vi "运维调试_采配水_古田户外.vi"() -> ()   [LabVIEW 2016, in "PLC.lvlib"]
uses:
  PLC.lvlib
  <vilib>/Plasmionique/MB Master/MB_Master/MB_Master.lvclass
  <vilib>/Utility/miscctls.llb/LVPointTypeDef.ctl
  <vilib>/Plasmionique/MB Master/MB_Master_Serial/MB_Master_Serial.lvclass
  D:/Program Files (x86)/National Instruments/LabVIEW 2016/vi.lib/Plasmionique/MB Master/MB_Master/MB_Master.lvclass
  <vilib>/Plasmionique/MB Master/MB Master.lvlib
panel:
  out "Y7":bool caption="V6 空压机"
  out "Y6":bool caption="V5 排液阀"
  out "Y5":bool caption="V4 二级清洗阀"
  out "Y4":bool caption="V3 一级清洗阀"
  out "Y3":bool caption="V2 外部管路清洗阀"
  out "Y2":bool caption="M2 增压泵"
  out "Y1":bool caption="V1 进样阀"
  out "Y0":bool caption="M1 潜水泵"
  out "X7":bool caption="采水泵过载检测"
  out "X6":bool caption="断电检测"
  out "X5":bool caption="开门检测"
  out "X4":bool caption="烟雾检测"
  out "X3":bool caption="漏水检测"
  out "X2":bool caption="进样检测"
  out "X1":bool
  out "X0":bool caption="采样池液位开关"
  out "R109":i16 caption="配水时间"
  out "集成报警信息":string
  out "R108":i16 caption="自来水报警"
  out "R107":i16 caption="采水池液位报警设置"
  out "R106":i16 caption="进样超时设置"
  out "R105":i16 caption="二级清洗时间"
  out "R104":i16 caption="一级清洗时间"
  out "R103":i16 caption="外部管路清洗时间"
  out "R102":i16 caption="静置沉淀时间"
  out "R101":i16 caption="内部管路润洗时间"
  out "R100":i16 caption="外部管路润洗时间"
  out "R2":i16
  out "R1":i16
  out "多列列表框":i32(listbox)
  out "R19":i16
  out "R18":i16
  out "R17":i16
  out "R16":i16
  out "R15":i16
  out "R14":i16
  out "R13":i16
  out "R12":i16
  in  "V6":bool
  in  "V5":bool
  in  "V4":bool
  in  "V3":bool
  in  "V2":bool
  in  "M2":bool
  in  "V1":bool
  in  "M1":bool
  in  "返回":bool
  in  "参数设置":bool
  in  "单步启动":bool
  in  "启动":bool
  in  "停止":bool
  # "S"
  # "S"
  # "S"
  # "S"
  # "S"
  # "S"
  # "S"
  # "S"
  # "S"
  # "S"
  # "单步计时："
  # "s"
  # "流程计时："
  # "s"
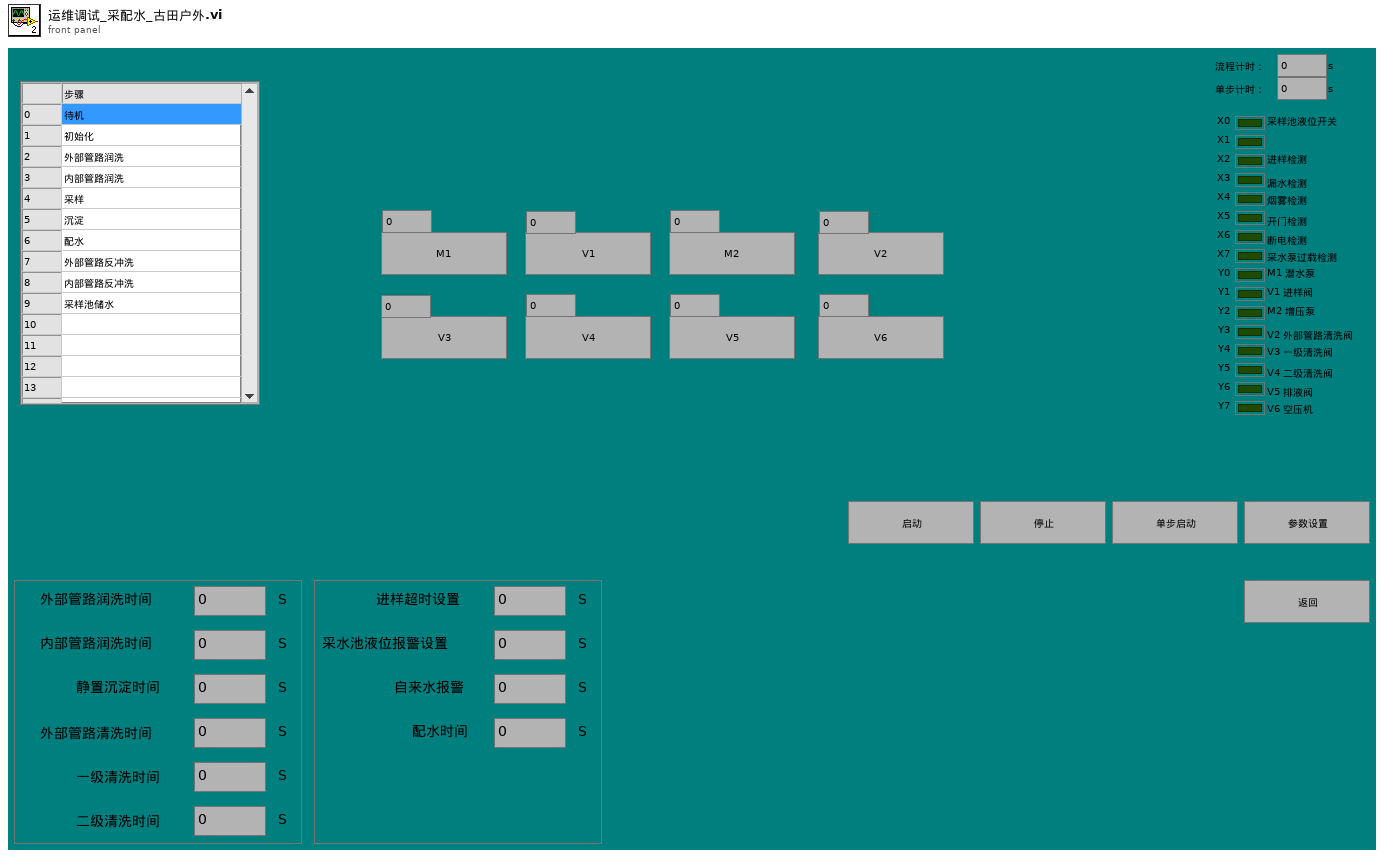
[diagram p1: front panel]
types:
  T1 = typedef "LVPointTypeDef.ctl" = cluster{"Horizontal":i16, "Vertical":i16}
  T2 = cluster{"时间标识":timestamp, "设备":string, "日志信息":string}
  T3 = cluster{"R0":i16, "R1":i16, "R2":i16, "R3":i16, "R4":i16, "R5":i16, "R6":i16, "R7":i16, "R8":i16, "R9":i16, "R10":i16, "R11":i16, "R12":i16, "R13":i16, "R14":i16, "R15":i16, "R16":i16, "R17":i16, "R18":i16, "R19":i16}
  T4 = cluster{"coil values[0]":bool, "coil values[1]":bool, "coil values[2]":bool, "coil values[3]":bool, "coil values[4]":bool, "coil values[5]":bool, "coil values[6]":bool, "coil values[7]":bool, "coil values[8]":bool, "coil values[9]":bool, "coil values[10]":bool, "coil values[11]":bool, "coil values[12]":bool, "coil values[13]":bool, "coil values[14]":bool, "coil values[15]":bool}
  T5 = cluster{"seconds since 1Jan1904":timestamp, "table输入":string, string, "table输入":string}
  T6 = cluster{"时间标识":timestamp, "设备":string, "日志信息":string, "流程参数":string}
  T7 = cluster{"命令":string, cluster{"starting address":u16, "holding register value":u16}}
  T8 = enum16{"水样测量", "标样核查", "零点核查", "加标回收", "平行样", "校零", "校标"}
  T9 = cluster{"是否启用仪器":bool, "CODMn":cluster{"启动测量模式":cluster{"测量模式":enum16{"水样测量", "标样核查", "零点核查", "加标回收", "平行样", "校零", "校标"}}, "确定按钮":bool}}
  T10 = cluster{"命令":string, "数据":cluster{"starting address":u16, "holding register value":u16}}
  T11 = cluster{"命令":string, "数据":cluster{"starting address":u16, "holding register values":u16[]}}
  T12 = cluster{"命令":string, "data":cluster{"starting address":u16, "coil values":bool[]}}
  T13 = enum32{"Bad", "Idle", "Run top level", "Running"}
  T14 = cluster{"baud rate (bps)":u32, "stop bits":u16, "parity":u16, "flow control":u16, "timeout":u32, "retries":i32}
  T15 = cluster{"starting address":u16, "holding register values":u16[]}
  T16 = cluster{"starting address":u16, "holding register value":u16}
  T17 = cluster{"starting address":u16, "coil values":bool[]}
  T18 = cluster{"Registers[0]":u16, "Registers[1]":u16, "Registers[2]":u16, "Registers[3]":u16, "Registers[4]":u16, "Registers[5]":u16, "Registers[6]":u16, "Registers[7]":u16, "Registers[8]":u16, "Registers[9]":u16, "Registers[10]":u16, "Registers[11]":u16, "Registers[12]":u16, "Registers[13]":u16, "Registers[14]":u16, "Registers[15]":u16, "Registers[16]":u16, "Registers[17]":u16, "Registers[18]":u16, "Registers[19]":u16}
  T19 = cluster{"Registers[0]":u16, "Registers[1]":u16, "Registers[2]":u16, "Registers[3]":u16, "Registers[4]":u16, "Registers[5]":u16}
  T20 = cluster{"Coils[0]":bool, "Coils[1]":bool, "Coils[2]":bool, "Coils[3]":bool, "Coils[4]":bool, "Coils[5]":bool, "Coils[6]":bool, "Coils[7]":bool, "Coils[8]":bool, "Coils[9]":bool, "Coils[10]":bool, "Coils[11]":bool, "Coils[12]":bool, "Coils[13]":bool, "Coils[14]":bool, "Coils[15]":bool}
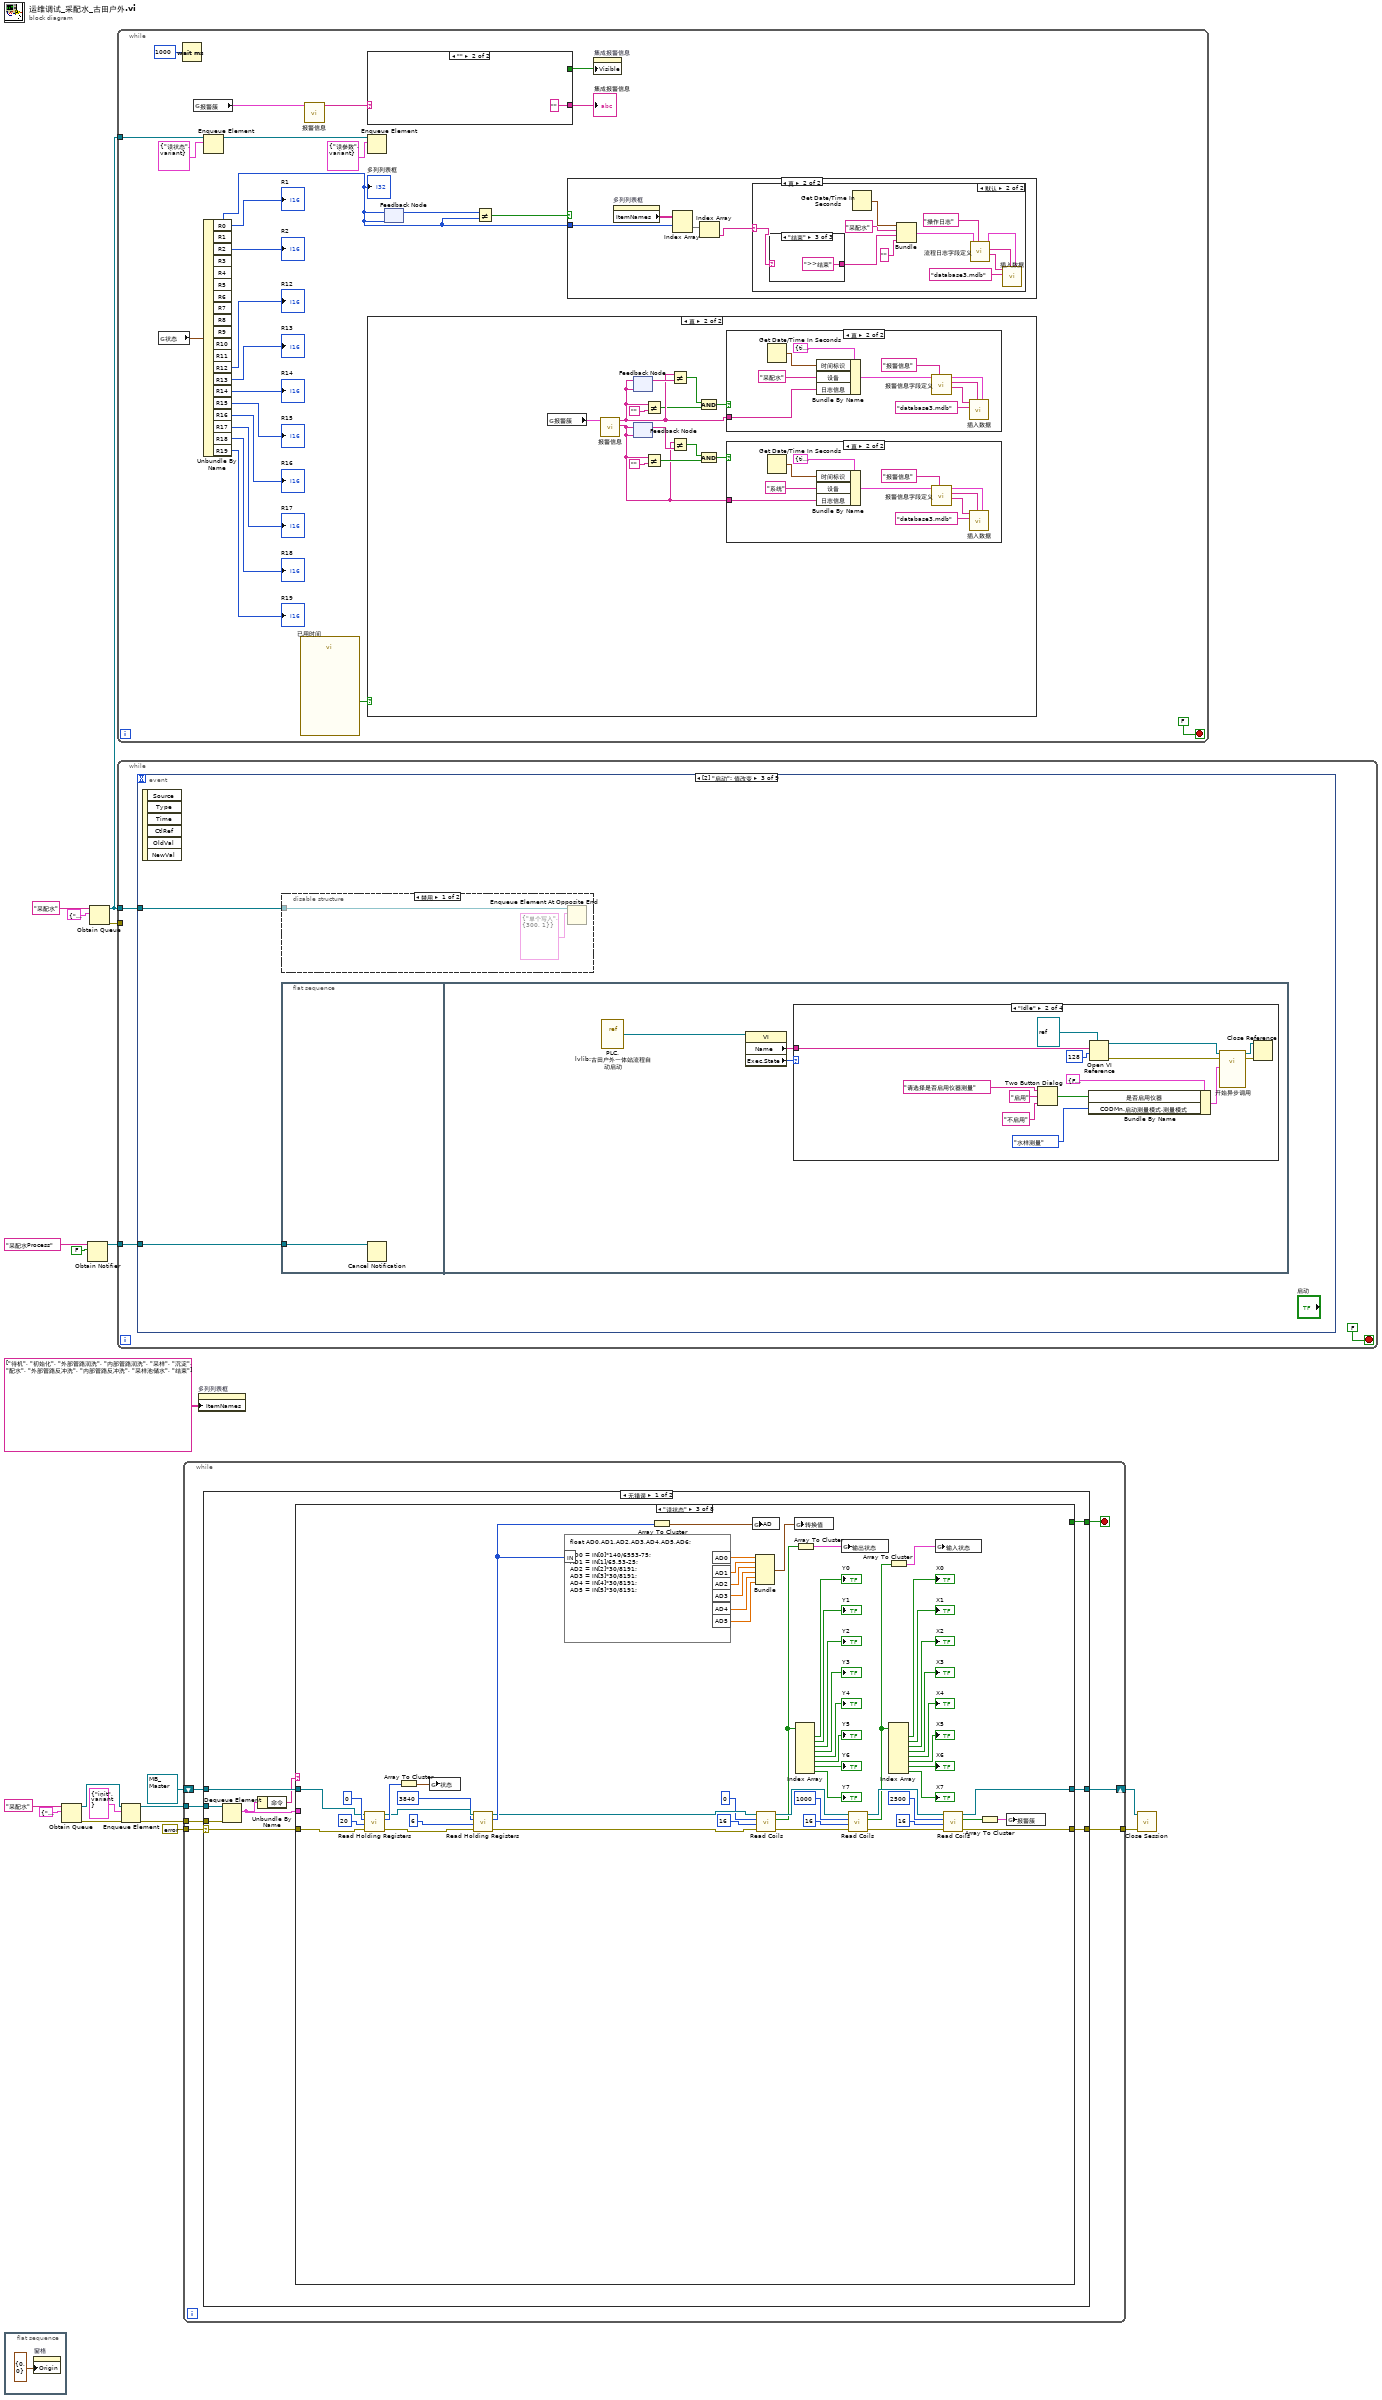
[diagram p0: block diagram]
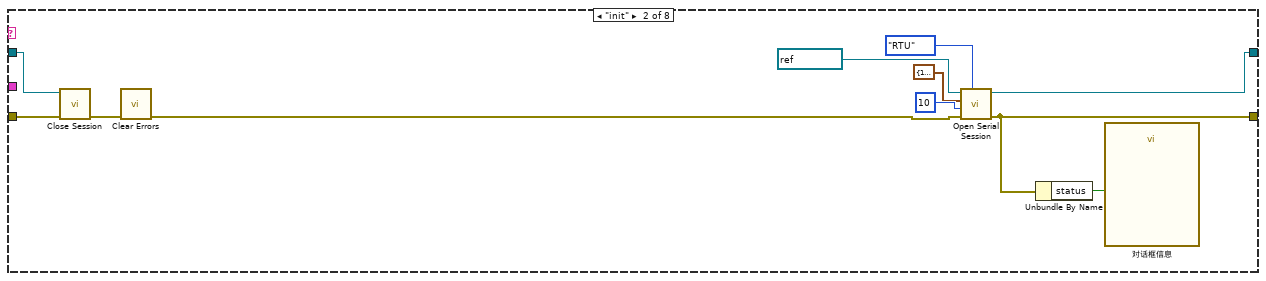
[diagram p3: hidden frame]
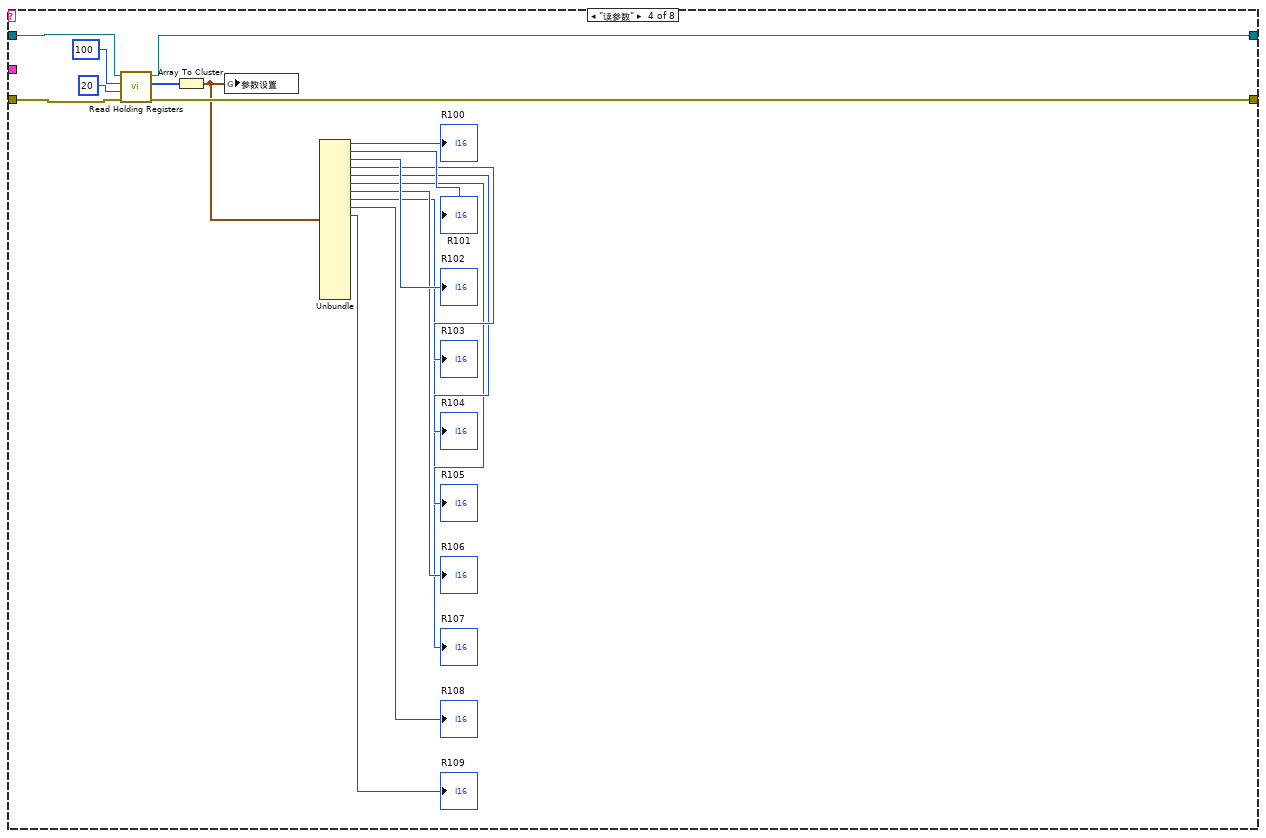
[diagram p4: hidden frame]
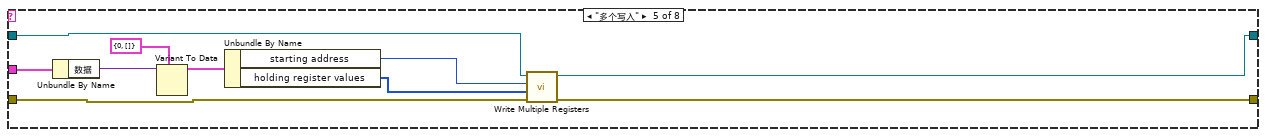
[diagram p5: hidden frame]
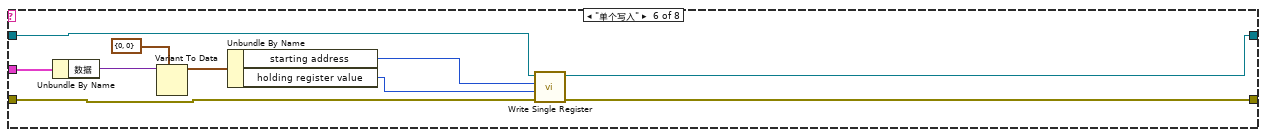
[diagram p6: hidden frame]
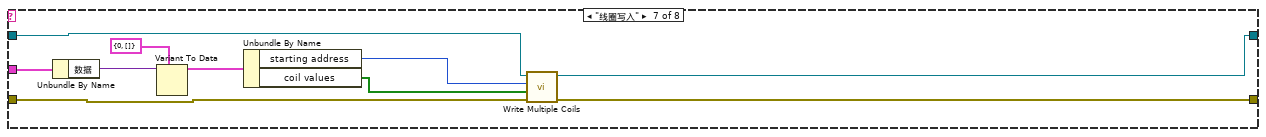
[diagram p7: hidden frame]
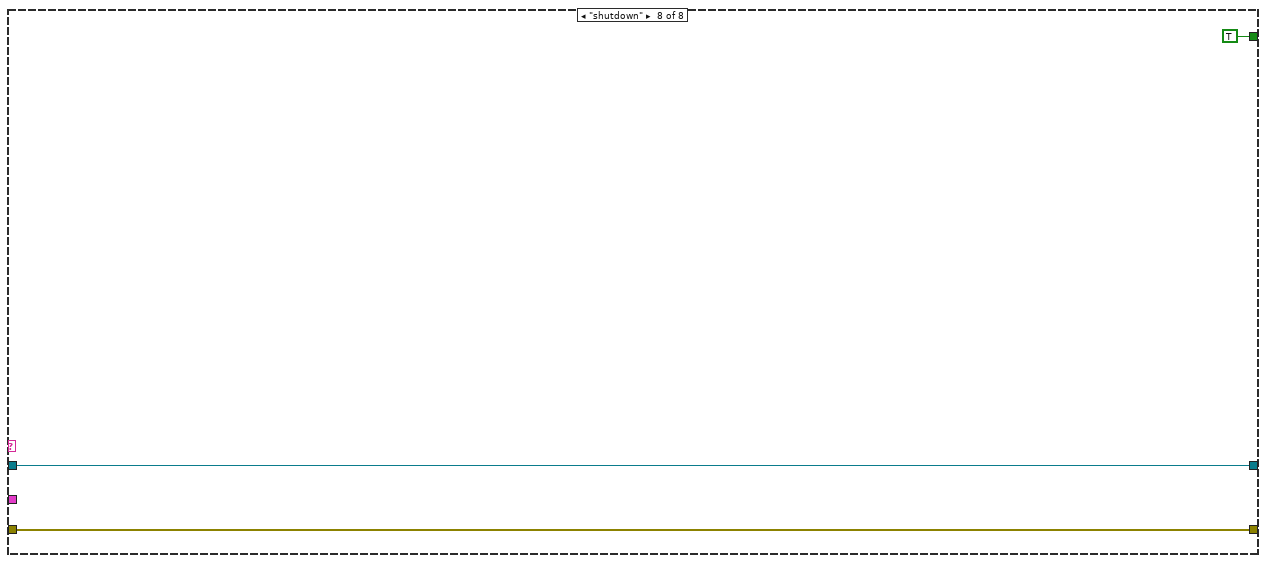
[diagram p8: hidden frame]
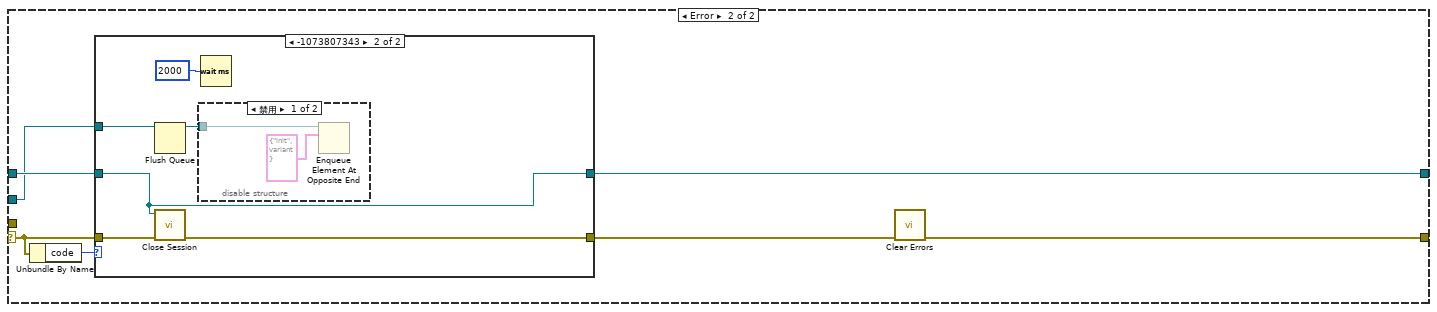
[diagram p9: hidden frame]
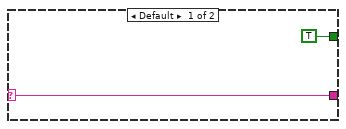
[diagram p15: hidden frame]
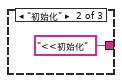
[diagram p19: hidden frame]
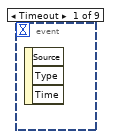
[diagram p20: hidden frame]
diagram:
  n1 = flat-sequence {
    frame #0 {
      n2 = property on="窗格" class="Pane"("Origin"=T1 {"Horizontal"=0, "Vertical"=0} ("原点")) -> ()  [unwired: 2 in, 2 out]
    }
  }
  n3 = Obtain Queue(name (unnamed)="采配水" ("名称（未命名）"), element data type=cluster{"命令":string, "数据":variant} {"命令"="", "数据"=variant}) -> (queue out=w9:refnum<queue>, error out=w8:errorcluster)  [unwired: 3 in, 1 out]
  n4 = Obtain Notifier(name (unnamed)="采配水Process" ("名称（未命名）"), notification data type=FALSE) -> (notifier out=w12:refnum<notifier>)  [unwired: 2 in, 2 out]
  n5 = Obtain Queue(name (unnamed)="采配水" ("名称（未命名）"), element data type=cluster{"命令":string, "数据":variant} {"命令"="", "数据"=variant}) -> (queue out=w16:refnum<queue>, error out=w17:errorcluster)  [unwired: 3 in, 1 out]
  n6 = while {
    tunnel: w16 -> [w44]
    stop <- FALSE stop-if-true
    n7 = global read "采配水全局变量.vi" "状态"() -> (w42:T3)
    n8 = Wait (ms)(milliseconds to wait=u32 1000 ("等待时间（毫秒）")) -> ()  [unwired: 1 out]
    n9 = global read "采配水全局变量.vi" "报警簇"() -> (w30:T4)
    n10 = Unbundle By Name(w42) -> ("R0"=w22:i16, "R1"=→"R1":i16, "R2"=→"R2":i16, "R12"=→"R12":i16, "R13"=→"R13":i16, "R14"=→"R14":i16, "R15"=→"R15":i16, "R16"=→"R16":i16, "R17"=→"R17":i16, "R18"=→"R18":i16, "R19"=→"R19":i16)  [unwired: 9 out]
    "多列列表框" <- w22
    n11 = Enqueue Element(queue=w44, element=cluster{"命令":string, "数据":variant} {"命令"="读状态", "数据"=variant} ("元素")) -> (queue out=w24:refnum<queue>)  [unwired: 2 in, 2 out]
    n12 = call "已用时间"() -> ("Time has Elapsed"=w27:bool)  [unwired: 12 in, 7 out]
    n13 = call "报警信息.vi"("报警簇"=w30) -> ("采配水报警信息"=w21:string)  [unwired: 9 in, 1 out]
    n14 = case shown="\"\"" w21 {
      selector: w21 -> [w80 _]
      tunnel: [w80 "" ("字符串")] -> w29
      tunnel: [TRUE ("可见") _] -> w28
      frame Default {
      }
      frame "" {
      }
    }
    "集成报警信息" <- w29
    n15 = Enqueue Element(queue=w24, element=cluster{"命令":string, "数据":variant} {"命令"="读参数", "数据"=variant} ("元素")) -> ()  [unwired: 2 in, 3 out]
    n16 = case shown="真" w27 {
      frame False {
      }
      frame True {
        n17 = global read "采配水全局变量.vi" "报警簇"() -> (w58:T4)
        n18 = call "报警信息.vi"("报警簇"=w58) -> ("系统报警信息"=w47:string, "采配水报警信息"=w54:string)  [unwired: 9 in]
        n19 = feedback #1(w54) -> (w57:string)
        n20 = feedback-in #1(w54) -> ()
        n21 = feedback #2(w47) -> (w48:string)
        n22 = feedback-in #2(w47) -> ()
        n23 = Not Equal?(x=w54, y="") -> (x != y?=w52:bool)
        n24 = Not Equal?(x=w47, y="") -> (x != y?=w51:bool)
        n25 = Not Equal?(x=w54, y=w57) -> (x != y?=w56:bool)
        n26 = Not Equal?(x=w47, y=w48) -> (x != y?=w49:bool)
        n27 = And(x=w56, y=w52) -> (x .and. y?=w55:bool)
        n28 = And(x=w49, y=w51) -> (x .and. y?=w46:bool)
        n29 = case shown="真" w55 {
          tunnel: w54 -> [_ w69]
          frame False {
          }
          frame True {
            n30 = Get Date/Time In Seconds() -> (seconds since 1Jan1904=w71:timestamp)
            n31 = Bundle By Name(cluster=T2 {"时间标识"=timestamp(0 s since 1904-01-01), "设备"="", "日志信息"=""} ("data in"), "时间标识"=w71, "设备"="采配水", "日志信息"=w69) -> (w72:T2)
            n32 = call "报警信息字段定义.vi"("table输入"="报警信息", "data in"=w72) -> ("table输出"=w76:string, "columns"=w77:string[], "data out"=w78:T2)  [unwired: 7 in]
            n33 = call "插入数据.vi"("data"=w78, "columns"=w77, "database"="database3.mdb", "table"=w76) -> ()  [unwired: 7 in, 1 out]
          }
        }
        n34 = case shown="真" w46 {
          tunnel: w47 -> [_ w59]
          frame False {
          }
          frame True {
            n35 = Get Date/Time In Seconds() -> (seconds since 1Jan1904=w61:timestamp)
            n36 = Bundle By Name(cluster=T2 {"时间标识"=timestamp(0 s since 1904-01-01), "设备"="", "日志信息"=""} ("data in"), "时间标识"=w61, "设备"="系统", "日志信息"=w59) -> (w62:T2)
            n37 = call "报警信息字段定义.vi"("table输入"="报警信息", "data in"=w62) -> ("table输出"=w66:string, "columns"=w67:string[], "data out"=w68:T2)  [unwired: 7 in]
            n38 = call "插入数据.vi"("data"=w68, "columns"=w67, "database"="database3.mdb", "table"=w66) -> ()  [unwired: 7 in, 1 out]
          }
        }
      }
    }
    n39 = feedback-in #3(w22) -> ()
    n40 = feedback #3(w22) -> (w23:i16)
    n41 = Not Equal?(x=w23, y=w22) -> (x != y?=w31:bool)
    n42 = case shown="真" w31 {
      tunnel: w22 -> [_ w84]
      frame False {
      }
      frame True {
        n43 = property on="多列列表框" class="MCListbox (严格)"() -> ("ItemNames"=w85:string[][])  [unwired: 2 in, 2 out]
        n44 = Index Array(array=w85, index (row)=w84) -> (element=w83:string[])  [unwired: 1 in]
        n45 = Index Array(array=w83) -> (element=w82:string)  [unwired: 1 in]
        n46 = case shown="默认" w82 {
          selector: w82 -> [_ w87]
          frame "待机" {
          }
          frame Default {
            n47 = case shown="\"结束\"" w87 {
              selector: w87 -> [w97 _ _]
              tunnel: [w97 "<<初始化" ">>结束"] -> w86
              frame Default {
              }
              frame "初始化" {
              }
              frame "结束" {
              }
            }
            n48 = Get Date/Time In Seconds() -> (seconds since 1Jan1904=w91:timestamp)
            n49 = Bundle("seconds since 1Jan1904"=w91, "table输入"="采配水", w86, "table输入"="") -> (w89:T5)  [unwired: 1 in]
            n50 = call "流程日志字段定义.vi"("table输入"="操作日志", "data in"=w89) -> ("table输出"=w94:string, "columns"=w95:string[], "data out"=w96:T6)  [unwired: 7 in]
            n51 = call "插入数据.vi"("data"=w96, "columns"=w95, "database"="database3.mdb", "table"=w94) -> ()  [unwired: 7 in, 1 out]
          }
        }
      }
    }
    n52 = property on="集成报警信息" class="Str"("Visible"=w28) -> ()  [unwired: 2 in, 2 out]
  }
  n53 = while {
    tunnel: w16 -> [w101]
    tunnel: w17 -> [_]
    tunnel: w12 -> [w100]
    stop <- FALSE stop-if-true
    n54 = event shown="[2] \"启动\": 值改变" {
      selector: _ -> [_ _ _ _ _ _ _ _ _]
      dyn-events: _ -> [_ _ _ _ _ _ _ _ _]
      timeout: _ -> [_ _ _ _ _ _ _ _ _]
      tunnel: w101 -> [_ w105 w108 w133 w148 _ _ _ w166]
      tunnel: w100 -> [_ w104 w107 _ _ _ _ _ _]
      event Timeout {
        n55 = event-data() -> ()  [unwired: 1 in, 3 out]
      }
      event "停止": Value Change {
        n56 = event-data() -> ()  [unwired: 1 in, 6 out]
        n57 = Send Notification(notification=TRUE ("通知"), notifier=w104) -> ()  [unwired: 1 in, 2 out]
        n58 = Enqueue Element At Opposite End(queue=w105, element=T7 {"命令"="单个写入", {"starting address"=300, "holding register value"=2}} ("元素")) -> ()  [unwired: 2 in, 3 out]
      }
      event "启动": Value Change {
        n59 = event-data() -> ()  [unwired: 1 in, 6 out]
        n60 = disable-structure shown="禁用" {
          disable-tunnel: w108 -> [w129 _]
          frame Disabled {
            n61 = Enqueue Element At Opposite End(queue=w129, element=T7 {"命令"="单个写入", {"starting address"=300, "holding register value"=1}} ("元素")) -> ()  [unwired: 2 in, 3 out]
          }
          frame Enabled {
          }
        }
        n62 = flat-sequence {
          tunnel: w107 -> [w109]
          frame #0 {
            n63 = Cancel Notification(0:w109) -> ()  [unwired: 1 in, 3 out]
          }
          frame #1 {
            n64 = vi-ref "PLC.lvlib:古田户外一体站流程自动启动.vi"() -> (w112:refnum<vi>)
            n65 = property class="VI"(reference=w112) -> ("Name"=w111:string, "Exec.State"=w110:T13)  [unwired: 1 in, 2 out]
            n66 = case shown="\"Idle\"" w110 {
              tunnel: w111 -> [_ w126 _ _]
              frame "Bad", Default {
              }
              frame "Idle" {
                n67 = Two Button Dialog(message="请选择是否启用仪器测量" ("消息"), 1:"不启用" ("F按钮名称（“取消”）"), 2:"启用" ("T按钮名称（“确定”）")) -> (T button?=w116:bool)
                n68 = Bundle By Name(cluster=T9 {"是否启用仪器"=FALSE, "CODMn"={"启动测量模式"={"测量模式"=enum."水样测量"}, "确定按钮"=FALSE}} ("参数"), "是否启用仪器"=w116, "CODMn.启动测量模式.测量模式"=T8."水样测量") -> (w113:T9)
                n69 = Open VI Reference(type specifier VI Refnum (for type only)=refnum<vi> refnum, vi path=w126, options=128 ("选项")) -> (vi reference=w124:refnum<vi>, error out=w121:errorcluster)  [unwired: 3 in]
                n70 = call-by-ref "开始异步调用"(reference=w124, error in=w121, "参数"=w113) -> (reference out=w122:refnum<vi>, error out=w120:errorcluster)  [unwired: 11 in]
                n71 = Close Reference(reference=w122, error in (no error)=w120) -> ()  [unwired: 1 out]
              }
              frame "Run top level" {
              }
              frame "Running" {
                n72 = One Button Dialog(message="流程已经运行,无须重复启动" ("消息")) -> ()  [unwired: 1 in, 1 out]
              }
            }
          }
        }
      }
      event "单步启动": Value Change {
        n73 = event-data() -> ()  [unwired: 1 in, 6 out]
        n74 = call "单步启动对话框.vi"() -> ("单步启动步骤输出"=w130:u16)  [unwired: 11 in]
        n75 = Bundle By Name(cluster=T10 {"命令"="单个写入", "数据"={"starting address"=301, "holding register value"=0}} ("元素"), "数据.holding register value"=w130) -> (w131:T10)
        n76 = Enqueue Element At Opposite End(queue=w133, element=w131) -> ()  [unwired: 2 in, 3 out]
      }
      event "R100", "R101", "R102", "R103", "R104", "R105", "R106", "R107", "R108", "R109": Value Change {
        n77 = event-data() -> ()  [unwired: 1 in, 6 out]
        n78 = local read "R100"() -> (w143:i16)
        n79 = local read "R101"() -> (w142:i16)
        n80 = local read "R102"() -> (w141:i16)
        n81 = local read "R103"() -> (w140:i16)
        n82 = local read "R104"() -> (w139:i16)
        n83 = local read "R105"() -> (w138:i16)
        n84 = local read "R106"() -> (w137:i16)
        n85 = local read "R107"() -> (w136:i16)
        n86 = local read "R108"() -> (w135:i16)
        n87 = local read "R109"() -> (w134:i16)
        n88 = Build Array(w143, w142, w141, w140, w139, w138, w137, w136, w135, w134) -> (w144:i16[])
        n89 = Bundle By Name(cluster=T11 {"命令"="多个写入", "数据"={"starting address"=0, "holding register values"=[]}} ("元素"), "数据.starting address"=u16 100, "数据.holding register values"=w144) -> (w145:T11)
        n90 = Enqueue Element At Opposite End(queue=w148, element=w145) -> ()  [unwired: 2 in, 3 out]
      }
      event "R100", "R101", "R102", "R103", "R104", "R105", "R106", "R107", "R108", "R109": Mouse Down {
        n91 = event-data() -> ("CtlRef"=w152:refnum<vi>)  [unwired: 1 in, 7 out]
        n92 = property class="DigNum (严格)"(reference=w152) -> (reference out=w150:refnum<vi>, "Value"=w151:i16)  [unwired: 1 in, 1 out]
        n93 = call "数字键盘.vi"("OldNumber"=w151) -> ("NewNumber"=w149:sgl)
        n94 = property class="DigNum (严格)"(reference=w150, "Val(Sgnl)"=w149) -> ()  [unwired: 1 in, 2 out]
      }
      event "参数设置": Value Change {
        n95 = event-data() -> ()  [unwired: 1 in, 6 out]
        n96 = property on="窗格" class="Pane"("Origin"=T1 {"Horizontal"=0, "Vertical"=528} ("原点")) -> ()  [unwired: 2 in, 2 out]
      }
      event "返回": Value Change {
        n97 = event-data() -> ()  [unwired: 1 in, 6 out]
        n98 = property on="窗格" class="Pane"("Origin"=T1 {"Horizontal"=0, "Vertical"=0} ("原点")) -> ()  [unwired: 2 in, 2 out]
      }
      event "M1", "V1", "M2", "V2", "V3", "V4", "V5", "V6": Value Change {
        n99 = event-data() -> ()  [unwired: 1 in, 6 out]
        n100 = Build Array("M1", "V1", "M2", "V2", "V3", "V4", "V5", "V6") -> (w155:bool[])
        n101 = Bundle By Name(cluster=T12 {"命令"="线圈写入", "data"={"starting address"=2400, "coil values"=[]}} ("元素"), "data.coil values"=w155) -> (w156:T12)
        n102 = Enqueue Element(queue=w166, element=w156) -> ()  [unwired: 2 in, 3 out]
      }
    }
  }
  n103 = Enqueue Element(queue=w9, element=cluster{"命令":string, "数据":variant} {"命令"="init", "数据"=variant} ("元素"), error in (no error)=w8) -> (queue out=w4:refnum<queue>, error out=w6:errorcluster)  [unwired: 1 in, 1 out]
  n104 = while {
    tunnel: w4 -> [w169]
    tunnel: w6 -> [w168]
    shift-right: [w173] -> w1
    shift-left: refnum<class "MB_Master.lvclass"> refnum ("MB session in") -> [w172]
    tunnel: errorcluster {"status"=FALSE, "code"=0, "source"=""} ("error out") -> [w170]
    tunnel: [w171] -> w2
    stop <- w167 stop-if-true
    n105 = case shown="无错误" w170 {
      selector: w170 -> [w179 w306]
      tunnel: [w182 w305] -> w173
      tunnel: w172 -> [w181 w307]
      tunnel: [w180 w303] -> w171
      tunnel: w169 -> [w176 w302]
      tunnel: w168 -> [w175 _]
      tunnel: [w177 _] -> w167
      frame No Error {
        n106 = Dequeue Element(queue=w176, error in (no error)=w175) -> (element=w174:cluster{"命令":string, "数据":variant})  [unwired: 1 in, 3 out]
        n107 = Unbundle By Name(w174) -> ("命令"=w178:string)
        n108 = case shown="\"读状态\"" w178 {
          tunnel: [w184 w188 w215 w263 w275 w285 w295 w300] -> w182
          tunnel: w181 -> [w184 w192 w235 w268 w278 w288 w298 w300]
          tunnel: [w183 w190 w214 w262 w276 w286 w296 w299] -> w180
          tunnel: w179 -> [w183 w194 w238 w267 w277 w287 w297 w299]
          tunnel: [_ _ _ _ _ _ _ TRUE] -> w177
          tunnel: w174 -> [_ _ _ _ w274 w284 w294 _]
          frame "idle", Default {
          }
          frame "init" {
            n109 = call-dynamic "Close Session.vi"("error in (no error)"=w194, "MB session in"=w192) -> ("error out"=w193:errorcluster)  [unwired: 9 in]
            n110 = call <vilib>:"Clear Errors.vi"("error in (no error)"=w193) -> ("error out"=w191:errorcluster)  [unwired: 5 in, 1 out]
            n111 = call <vilib>:"Open Serial Session.vi"("Mode (RTU)"=enum16{"RTU", "ASCII"}."RTU", "Error in"=w191, "Slave ID"=u8 10, "Serial Config"=T14 {"baud rate (bps)"=115200, "stop bits"=10, "parity"=0, "flow control"=0, "timeout"=1000, "retries"=1}, "VISA Resource"=refnum<visa-resource-name> "COM2" ("VISA resource name")) -> ("Error out"=w190:errorcluster, "MB_Serial session"=w188:refnum<class "MB_Master_Serial.lvclass">)  [unwired: 5 in]
            n112 = Unbundle By Name(w190) -> ("status"=w195:bool)
            n113 = call "对话框信息"("Enable"=w195) -> ()  [unwired: 9 in, 2 out]
          }
          frame "读状态" {
            n114 = call <vilib>:"Read Holding Registers.vi"("error in (no error)"=w238, "quantity"=u16 20 ("number of holding registers"), "starting address"=u16 0, "MB session in"=w235) -> ("error out"=w231:errorcluster, "Registers"=w234:u16[], "MB session out"=w233:refnum<class "MB_Master.lvclass">)  [unwired: 5 in]
            n115 = Array To Cluster(array=w234) -> (cluster=w240:T18)
            n116 = global write "采配水全局变量.vi" "状态"(w240) -> ()
            n117 = call <vilib>:"Read Holding Registers.vi"("error in (no error)"=w231, "quantity"=u16 6 ("number of holding registers"), "starting address"=u16 3840, "MB session in"=w233) -> ("error out"=w227:errorcluster, "Registers"=w232:u16[], "MB session out"=w228:refnum<class "MB_Master.lvclass">)  [unwired: 5 in]
            n118 = formula code="float AD0,AD1,AD2,AD3,AD4,AD5,AD6;\n\nAD0 = IN[0]*140/6553-75;\nAD1 = IN[1]/65.53-25;\nAD2 = IN[2]*30/8191;\nAD3 = IN[3]*30/8191;\nAD4 = IN[4]*30/8191;\nAD5 = IN[5]*30/8191;"("IN"=w232) -> ("AD0"=w246:dbl, "AD1"=w245:dbl, "AD2"=w244:dbl, "AD3"=w243:dbl, "AD4"=w242:dbl, "AD5"=w241:dbl)
            n119 = Array To Cluster(array=w232) -> (cluster=w248:T19)
            n120 = global write "采配水全局变量.vi" "AD"(w248) -> ()
            n121 = Bundle(w246, w245, w244, w243, w242, w241) -> (w247:cluster{dbl, dbl, dbl, dbl, dbl, dbl})  [unwired: 1 in]
            n122 = call <vilib>:"Read Coils.vi"("error in (no error)"=w227, "quantity"=u16 16 ("number of coils"), "starting address"=u16 0, "MB session in"=w228) -> ("error out"=w223:errorcluster, "Coils"=w204:bool[], "MB session out"=w224:refnum<class "MB_Master.lvclass">)  [unwired: 5 in]
            n123 = global write "采配水全局变量.vi" "转换值"(w247) -> ()
            n124 = Index Array(array=w204) -> (element #1=→"Y0":bool, element #2=→"Y1":bool, element #3=→"Y2":bool, element #4=→"Y3":bool, element #5=→"Y4":bool, element #6=→"Y5":bool, element #7=→"Y6":bool, element #8=→"Y7":bool)  [unwired: 8 in]
            n125 = Array To Cluster(array=w204) -> (cluster=w249:T20)
            n126 = global write "采配水全局变量.vi" "输出状态"(w249) -> ()
            n127 = call <vilib>:"Read Coils.vi"("error in (no error)"=w223, "quantity"=u16 16 ("number of coils"), "starting address"=u16 1000, "MB session in"=w224) -> ("error out"=w219:errorcluster, "Coils"=w213:bool[], "MB session out"=w220:refnum<class "MB_Master.lvclass">)  [unwired: 5 in]
            n128 = Index Array(array=w213) -> (element #1=→"X0":bool, element #2=→"X1":bool, element #3=→"X2":bool, element #4=→"X3":bool, element #5=→"X4":bool, element #6=→"X5":bool, element #7=→"X6":bool, element #8=→"X7":bool)  [unwired: 8 in]
            n129 = Array To Cluster(array=w213) -> (cluster=w250:T20)
            n130 = global write "采配水全局变量.vi" "输入状态"(w250) -> ()
            n131 = call <vilib>:"Read Coils.vi"("error in (no error)"=w219, "quantity"=u16 16 ("number of coils"), "starting address"=u16 2500, "MB session in"=w220) -> ("error out"=w214:errorcluster, "Coils"=w216:bool[], "MB session out"=w215:refnum<class "MB_Master.lvclass">)  [unwired: 5 in]
            n132 = Array To Cluster(array=w216) -> (cluster=w239:T20)
            n133 = global write "采配水全局变量.vi" "报警簇"(w239) -> ()
          }
          frame "读参数" {
            n134 = call <vilib>:"Read Holding Registers.vi"("error in (no error)"=w267, "quantity"=u16 20 ("number of holding registers"), "starting address"=u16 100, "MB session in"=w268) -> ("error out"=w262:errorcluster, "Registers"=w264:u16[], "MB session out"=w263:refnum<class "MB_Master.lvclass">)  [unwired: 5 in]
            n135 = Array To Cluster(array=w264) -> (cluster=w251:T18)
            n136 = global write "采配水全局变量.vi" "参数设置"(w251) -> ()
            n137 = Unbundle(w251) -> ("Registers[0]"=→"R100":u16, "Registers[1]"=→"R101":u16, "Registers[2]"=→"R102":u16, "Registers[3]"=→"R103":u16, "Registers[4]"=→"R104":u16, "Registers[5]"=→"R105":u16, "Registers[6]"=→"R106":u16, "Registers[7]"=→"R107":u16, "Registers[8]"=→"R108":u16, "Registers[9]"=→"R109":u16)  [unwired: 10 out]
          }
          frame "多个写入" {
            n138 = Unbundle By Name(w274) -> ("数据"=w273:variant)
            n139 = Variant To Data(type=T15 {"starting address"=0, "holding register values"=[]}, Variant=w273) -> (data=w271:T15)  [unwired: 1 in, 1 out]
            n140 = Unbundle By Name(w271) -> ("starting address"=w270:u16, "holding register values"=w269:u16[])
            n141 = call <vilib>:"Write Multiple Registers.vi"("error in (no error)"=w277, "values"=w269, "starting address"=w270, "MB session in"=w278) -> ("error out"=w276:errorcluster, "MB session out"=w275:refnum<class "MB_Master.lvclass">)  [unwired: 6 in]
          }
          frame "单个写入" {
            n142 = Unbundle By Name(w284) -> ("数据"=w283:variant)
            n143 = Variant To Data(type=T16 {"starting address"=0, "holding register value"=0}, Variant=w283) -> (data=w281:T16)  [unwired: 1 in, 1 out]
            n144 = Unbundle By Name(w281) -> ("starting address"=w280:u16, "holding register value"=w279:u16)
            n145 = call <vilib>:"Write Single Register.vi"("error in (no error)"=w287, "value"=w279, "address"=w280, "MB session in"=w288) -> ("error out"=w286:errorcluster, "MB session out"=w285:refnum<class "MB_Master.lvclass">)  [unwired: 6 in]
          }
          frame "线圈写入" {
            n146 = Unbundle By Name(w294) -> ("数据"=w293:variant)
            n147 = Variant To Data(type=T17 {"starting address"=0, "coil values"=[]}, Variant=w293) -> (data=w291:T17)  [unwired: 1 in, 1 out]
            n148 = Unbundle By Name(w291) -> ("starting address"=w290:u16, "coil values"=w289:bool[])
            n149 = call <vilib>:"Write Multiple Coils.vi"("error in (no error)"=w297, "values"=w289, "starting address"=w290, "MB session in"=w298) -> ("error out"=w296:errorcluster, "MB session out"=w295:refnum<class "MB_Master.lvclass">)  [unwired: 6 in]
          }
          frame "shutdown" {
          }
        }
      }
      frame Error {
        n150 = Unbundle By Name(w306) -> ("code"=w308:i32)
        n151 = case shown="-1073807343" w308 {
          tunnel: w307 -> [w310 w314]
          tunnel: w306 -> [w309 w316]
          tunnel: [w309 w315] -> w304
          tunnel: [w310 w314] -> w305
          tunnel: w302 -> [_ w313]
          frame Default {
          }
          frame -1073807343 {
            n152 = Flush Queue(queue=w313) -> (queue out=w312:refnum<queue>)  [unwired: 1 in, 2 out]
            n153 = call-dynamic "Close Session.vi"("error in (no error)"=w316, "MB session in"=w314) -> ("error out"=w315:errorcluster)  [unwired: 9 in]
            n154 = disable-structure shown="禁用" {
              disable-tunnel: w312 -> [w317 _]
              frame Disabled {
                n155 = Enqueue Element At Opposite End(queue=w317, element=cluster{"命令":string, "数据":variant} {"命令"="init", "数据"=variant} ("元素")) -> ()  [unwired: 2 in, 3 out]
              }
              frame Enabled {
              }
            }
            n156 = Wait (ms)(milliseconds to wait=u32 2000 ("等待时间（毫秒）")) -> ()  [unwired: 1 out]
          }
        }
        n157 = call <vilib>:"Clear Errors.vi"("error in (no error)"=w304) -> ("error out"=w303:errorcluster)  [unwired: 5 in, 1 out]
      }
    }
  }
  n158 = property on="多列列表框" class="MCListbox (严格)"("ItemNames"=string[][] [["待机"], ["初始化"], ["外部管路润洗"], ["内部管路润洗"], ["采样"], ["沉淀"], ["配水"], ["外部管路反冲洗"], ["内部管路反冲洗"], ["采样池储水"], ["结束"]] ("项名")) -> ()  [unwired: 2 in, 2 out]
  n159 = call-dynamic "Close Session.vi"("error in (no error)"=w2, "MB session in"=w1) -> ()  [unwired: 9 in, 1 out]
